vi "_Parse Markdown Steps.vi"(11 "Variant":variant) -> (3 "Variant 2":variant)   [LabVIEW 2017, in "csmdoc.lvlib"]
uses:
  csmdoc.lvlib
  _Typedef/DocElement.ctl
  _tool/_file/csm-file-support.lvlib
  Communicable State Machine.lvlib
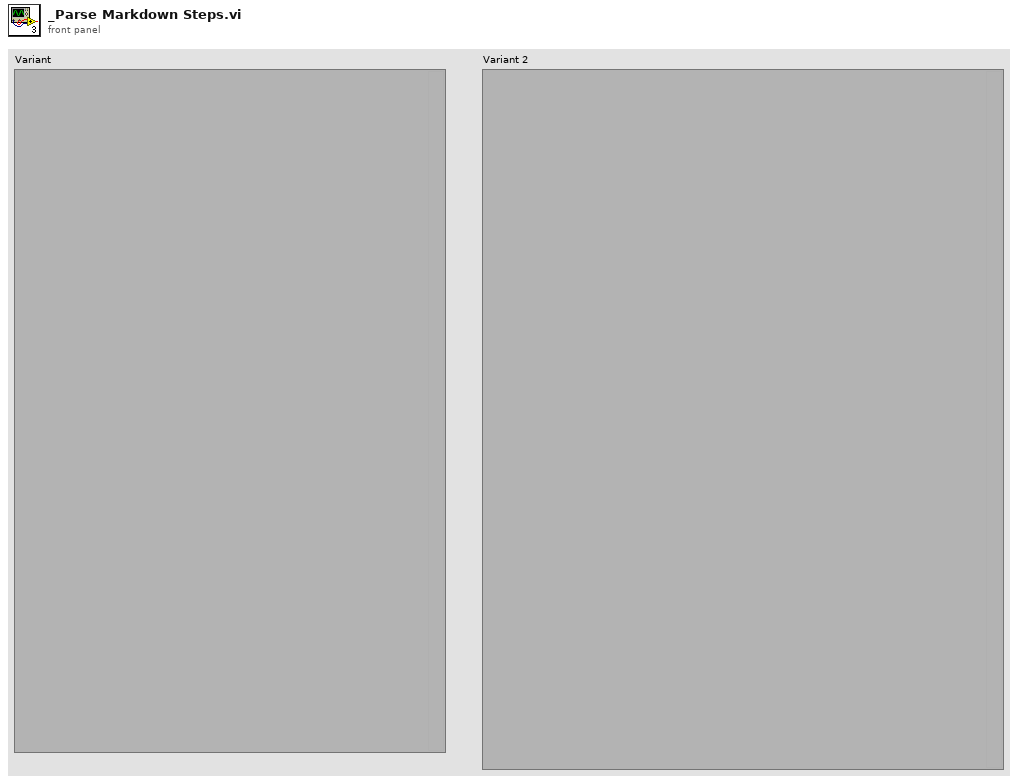
[diagram p1: front panel]
types:
  T1 = typedef "csmdoc.lvlib/DocElement.ctl" = cluster{"ID":string, "Content":string[], "SubIDs":string[], "Path":string[]}
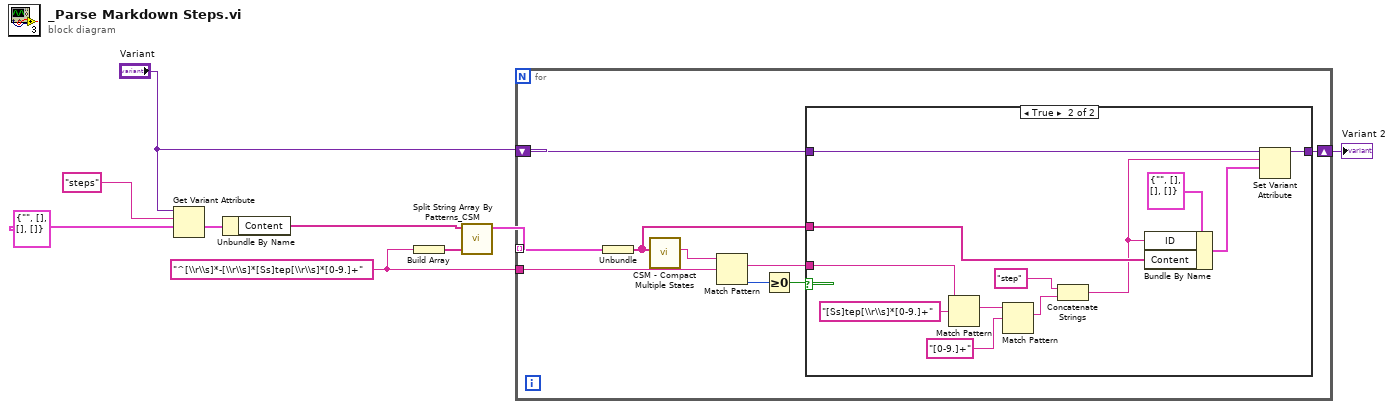
[diagram p0: block diagram]
diagram:
  w1 = "^[\\r\\s]*-[\\r\\s]*[Ss]tep[\\r\\s]*[0-9.]+" ("name")
  n1 = Get Variant Attribute(Variant="Variant", name="steps", default value (empty Variant)=T1 {"ID"="", "Content"=[], "SubIDs"=[], "Path"=[]} ("output cluster")) -> (value=w7:T1)  [unwired: 1 in, 3 out]
  n2 = Unbundle By Name(w7) -> ("Content"=w5:string[])
  n3 = Build Array(w1) -> (w6:string[])
  n4 = call "Split String Array By Patterns_CSM.vi"("Patterns"=w6, "Text Array"=w5) -> ("Array"=w4:cluster{"filtered array":string[]}[])  [unwired: 9 in]
  n5 = for {
    tunnel: w4 -> [w18] mode=indexing
    shift-right: [w15] -> w2
    shift-left: "Variant" -> [w16]
    tunnel: w1 -> [w10]
    n6 = Unbundle(w18) -> ("filtered array"=w12:string[])
    n7 = call "CSM - Compact Multiple States.vi"("Multiple States"=w12) -> ("States"=w17:string)  [unwired: 9 in]
    n8 = Match Pattern(string=w17, regular expression=w10) -> (match substring=w11:string, offset past match=w14:i32)  [unwired: 1 in, 2 out]
    n9 = Greater Or Equal To 0?(x=w14) -> (x >= 0?=w13:bool)
    n10 = case shown="True" w13 {
      tunnel: w16 -> [w19 w31]
      tunnel: [w19 w30] -> w15
      tunnel: w12 -> [_ w27]
      tunnel: w11 -> [_ w26]
      frame False {
      }
      frame True {
        n11 = Match Pattern(string=w26, regular expression="[Ss]tep[\\r\\s]*[0-9.]+") -> (match substring=w24:string)  [unwired: 1 in, 3 out]
        n12 = Match Pattern(string=w24, regular expression="[0-9.]+") -> (match substring=w22:string)  [unwired: 1 in, 3 out]
        n13 = Concatenate Strings("step" ("regular expression"), w22) -> (w20:string)
        n14 = Bundle By Name(cluster=T1 {"ID"="", "Content"=[], "SubIDs"=[], "Path"=[]} ("output cluster"), "ID"=w20, "Content"=w27) -> (w28:T1)
        n15 = Set Variant Attribute(Variant=w31, name=w20, value=w28) -> (Variant out=w30:variant)  [unwired: 1 in, 2 out]
      }
    }
  }
  "Variant 2" <- w2
